vi "Stop.vi"(8 "error in (no error)":errorcluster, 11 "ViewerRef":T1) -> (0 "error out":errorcluster)   [LabVIEW 2018, in "TopicViewer.lvlib"]
uses:
  TopicViewer.lvlib
  controls/viewewr_bus.ctl
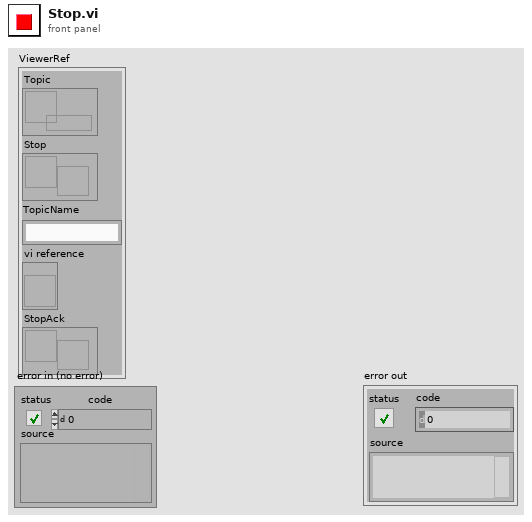
[diagram p1: front panel]
types:
  T1 = typedef "TopicViewer.lvlib/viewewr_bus.ctl" = cluster{"Topic":refnum<queue>, "Stop":refnum<notifier>, "TopicName":string, "vi reference":refnum<vi>, "StopAck":refnum<notifier>}
  T2 = enum32{"Bad", "Idle", "Run top level", "Running"}
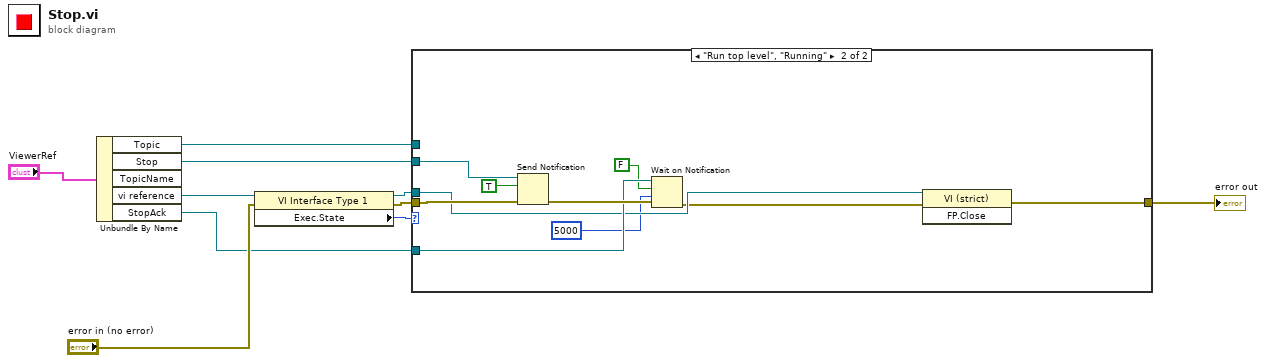
[diagram p0: block diagram]
diagram:
  n1 = Unbundle By Name("ViewerRef") -> ("Topic"=w4:refnum<queue>, "Stop"=w5:refnum<notifier>, "vi reference"=w9:refnum<vi>, "StopAck"=w1:refnum<notifier>)  [unwired: 1 out]
  n2 = property class="VI Interface Type 1"(reference=w9, error in="error in (no error)") -> (reference out=w3:refnum<vi>, error out=w6:errorcluster, "Exec.State"=w7:T2)
  n3 = case shown="\"Run top level\", \"Running\"" w7 {
    tunnel: w6 -> [w11 w20]
    tunnel: w5 -> [_ w21]
    tunnel: w4 -> [_ _]
    tunnel: w3 -> [_ w15]
    tunnel: [w11 w17] -> w2
    tunnel: w1 -> [_ w16]
    frame Default {
    }
    frame "Run top level", "Running" {
      n4 = Send Notification(notification=TRUE, notifier=w21, error in (no error)=w20) -> (error out=w19:errorcluster)  [unwired: 1 out]
      n5 = Wait on Notification(notifier=w16, ignore previous (F)=FALSE, timeout in ms (-1)=5000, error in (no error)=w19) -> (error out=w14:errorcluster)  [unwired: 3 out]
      n6 = invoke class="VI (strict)" method="FP.Close"(reference=w15, error in=w14) -> (error out=w17:errorcluster)  [unwired: 1 in, 2 out]
    }
  }
  "error out" <- w2
